vi "magnetic-actuator.vi"() -> ()   [LabVIEW 2021]
uses:
  mag-settings.ctl
panel:
  in  "On":bool
  in  "Off":bool
  out "Cycle Running":bool
  out "Last Command Sent":string
  out "Countdown Timer (mS)":u32
  out "last event":u32
  out "Coil Active":bool
  in  "Stop Cycle":bool
  in  "Start Cycle":bool
  in  "Eng Mode":bool
  out "LOW Cycle Time (Seconds)":dbl
  out "HIGH Cycle Time (Seconds)":dbl
  out "Duty %":dbl
  in  "Reflux Ratio":dbl
  in  "Period (Seconds)":dbl=5.0
  in  "Exit Program":bool
  # "TODO: CHANGE CYCLE TIME DISPLAY"
  # "TODO: MAKE THIS AESTHETIC"
  # "HIGH Cycle = period*(1/Duty Cycle)"
  # "Manual Controls"
  # "LOW Cycle = period - HIGH Cycle Time"
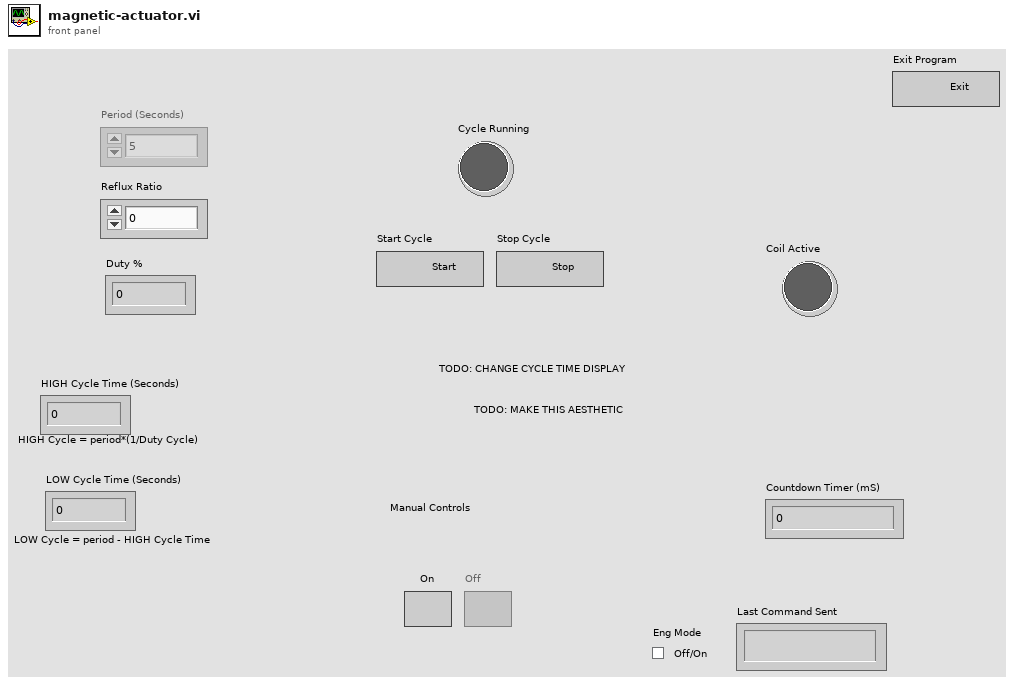
[diagram p1: front panel]
types:
  T1 = typedef "mag-settings.ctl" = cluster{"COM Port (COM10)":refnum<visa-resource-name>, "ADAM-ID":dbl, "ADAM-DO-channel":dbl, "Period (Seconds)":dbl, "Duty Cycle":dbl, "Eng Mode":bool}
  T2 = enum8{"Enabled", "Disabled", "Disabled and Grayed Out"}
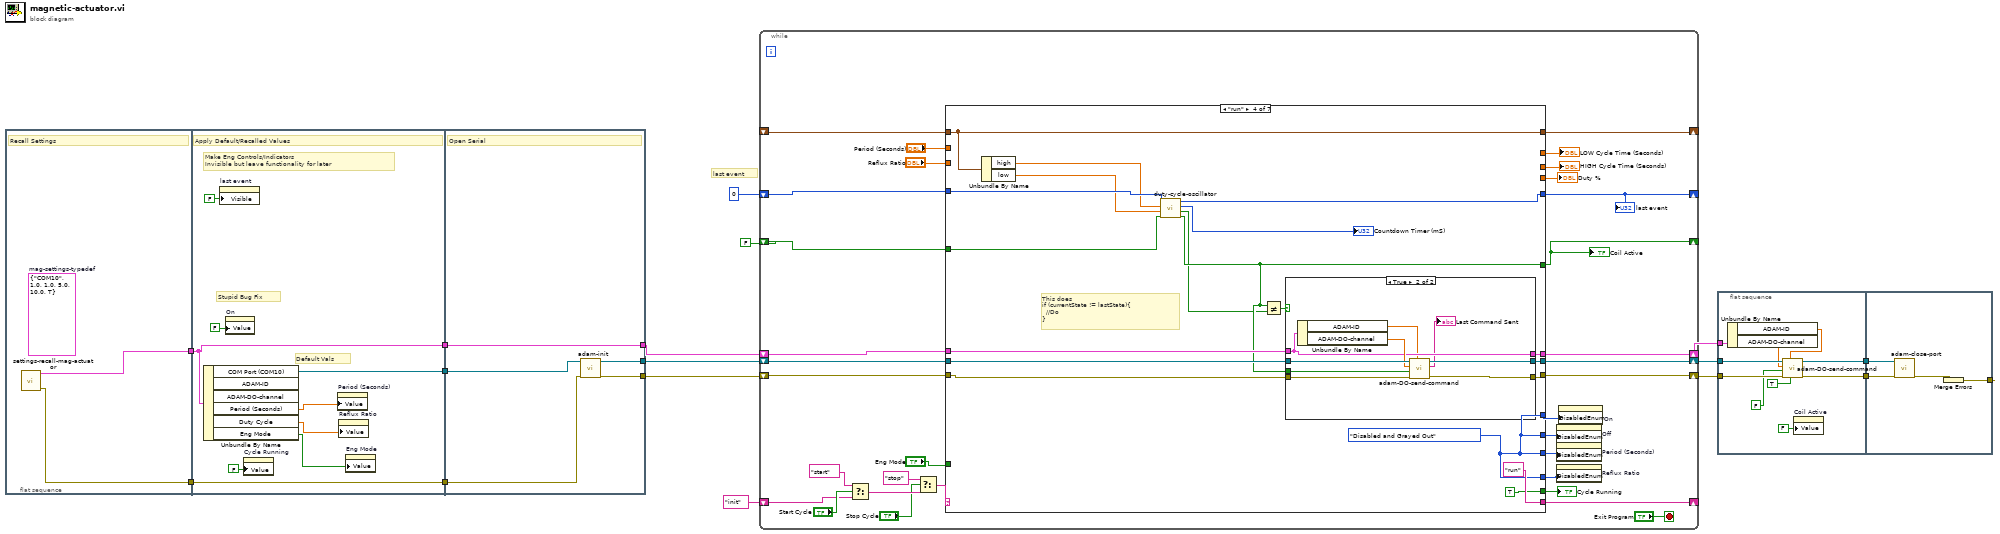
[diagram p0: block diagram]
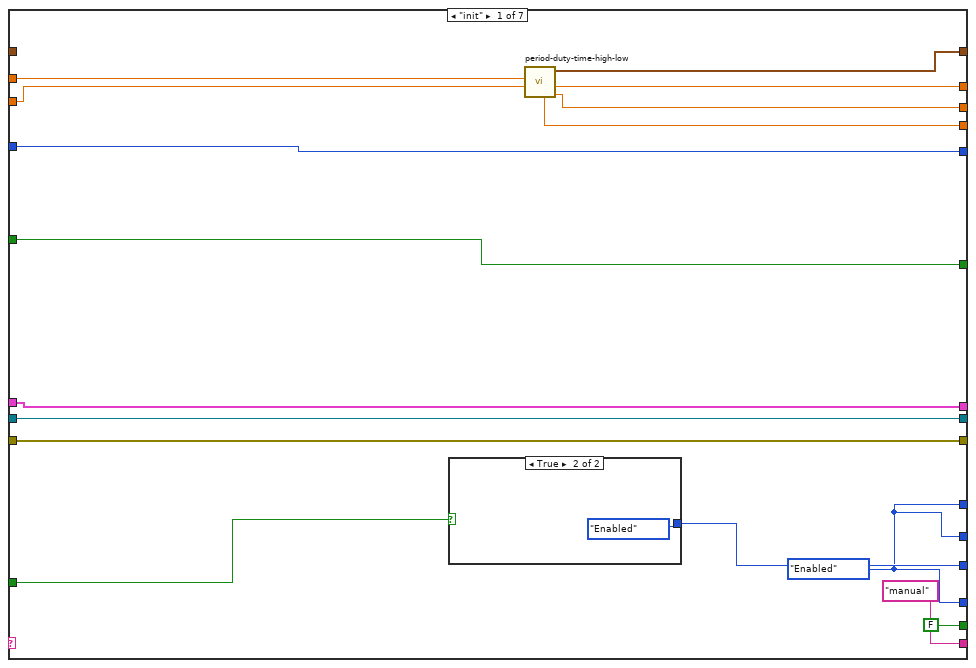
[diagram p2: hidden frame]
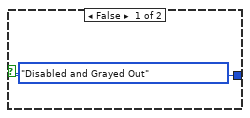
[diagram p3: hidden frame]
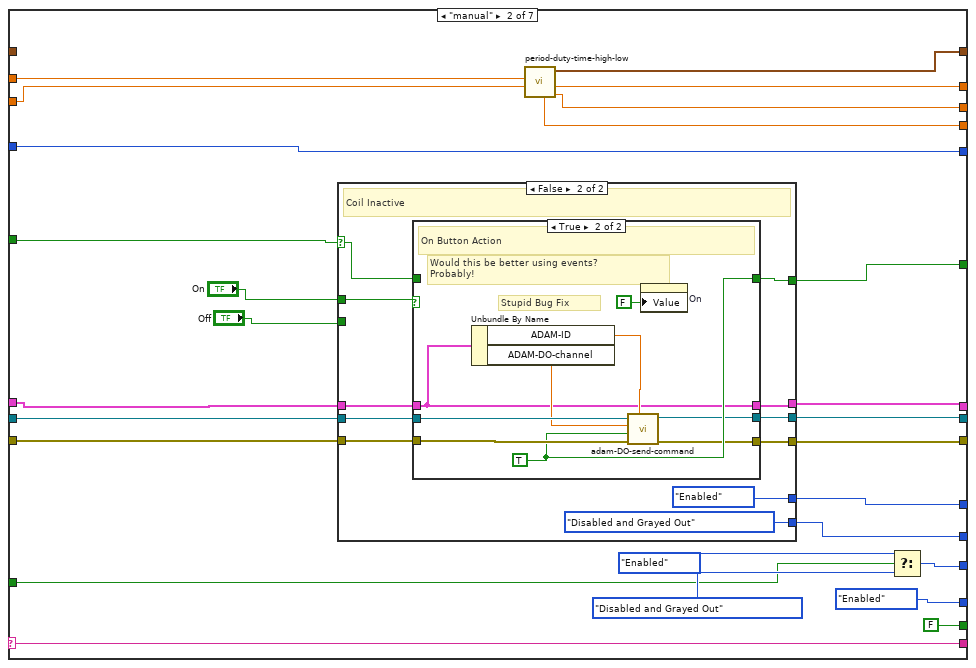
[diagram p4: hidden frame]
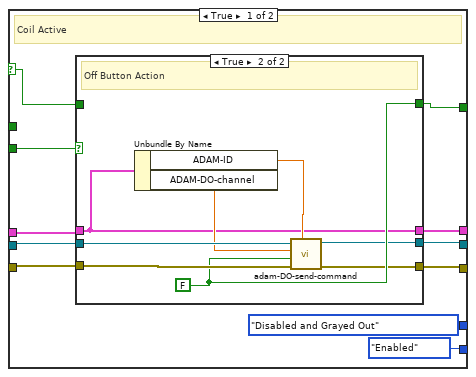
[diagram p5: hidden frame]
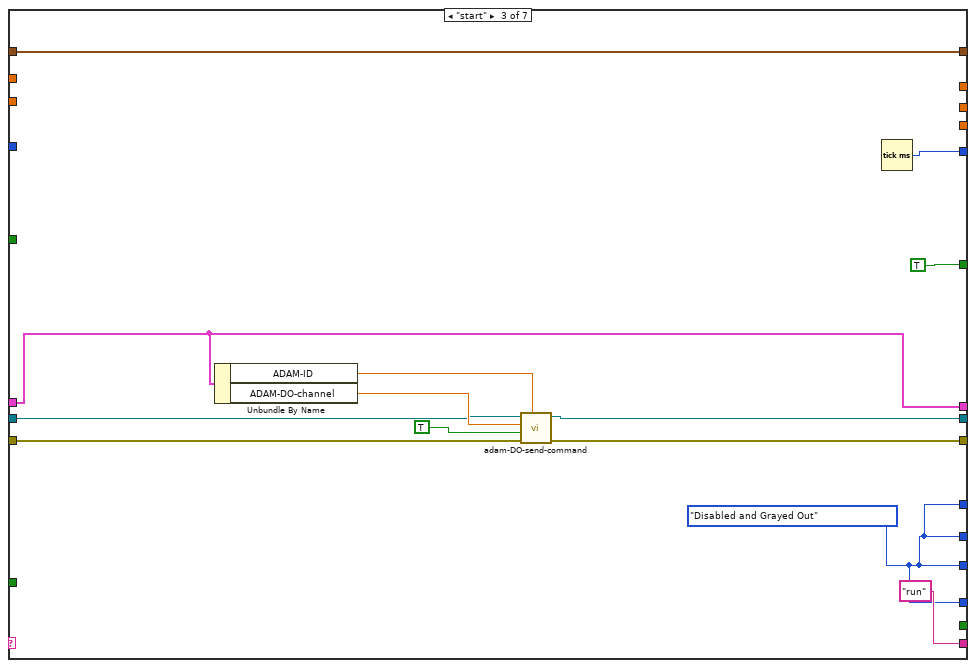
[diagram p8: hidden frame]
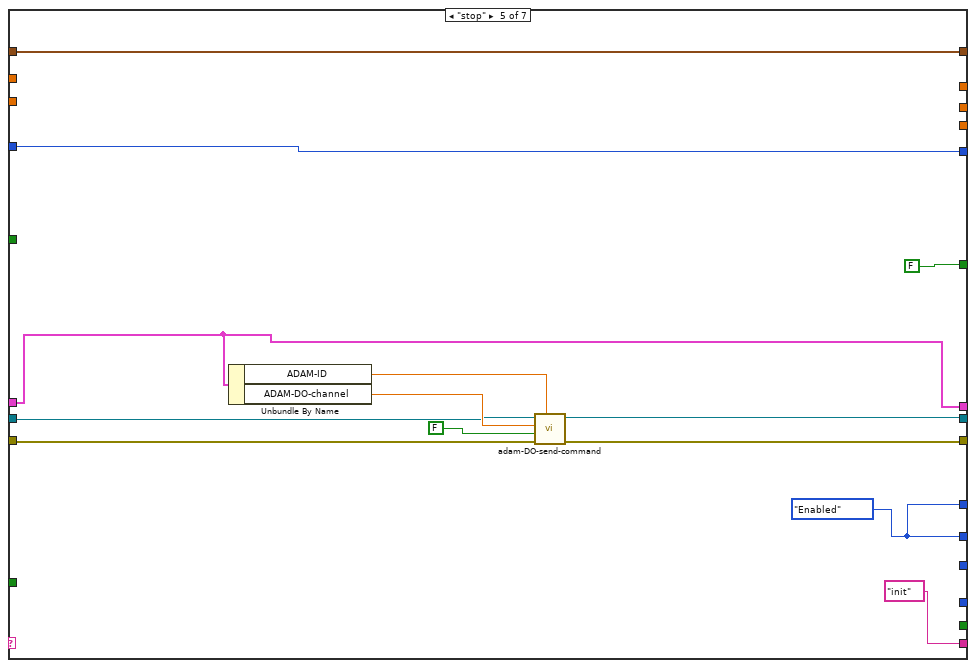
[diagram p10: hidden frame]
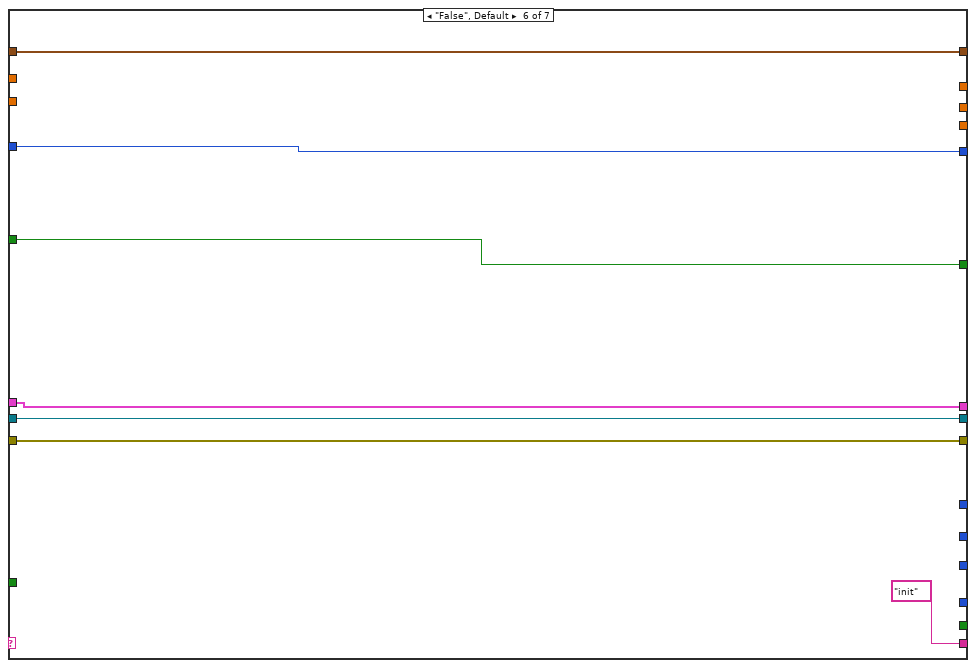
[diagram p11: hidden frame]
diagram:
  # "last event"
  n1 = flat-sequence {
    tunnel: [w18] -> w13
    tunnel: [w17] -> w5
    tunnel: [w27] -> w14
    tunnel: w13 -> [w26]
    tunnel: [w26] -> w12
    tunnel: w5 -> [w25]
    tunnel: [w25] -> w4
    tunnel: [w32] -> w11
    tunnel: [w31] -> w10
    tunnel: w14 -> [w29]
    tunnel: w12 -> [w30]
    tunnel: [w28] -> w3
    tunnel: w4 -> [w28]
    frame #0 {
      (unwired) T1 {"COM Port (COM10)"="COM10", "ADAM-ID"=1.0, "ADAM-DO-channel"=1.0, "Period (Seconds)"=5.0, "Duty Cycle"=10.0, "Eng Mode"=TRUE}  # mag-settings-typedef
      # "Recall Settings"
      n2 = call "settings-recall-mag-actuator.vi"() -> ("error out"=w18:errorcluster, "mag-settings"=w17:T1)  [unwired: 9 in, 1 out]
    }
    frame #1 {
      # "Default Vals"
      # "Make Eng Controls/Indicators\nInvisible but leave functionality for later"
      # "Stupid Bug Fix"
      # "Apply Default/Recalled Values"
      n3 = Unbundle By Name(w25) -> ("COM Port (COM10)"=w27:refnum<visa-resource-name>, "Period (Seconds)"=w24:dbl, "Duty Cycle"=w23:dbl, "Eng Mode"=w22:bool)  [unwired: 2 out]
      n4 = property on="last event" class="DigNum (strict)"("Visible"=FALSE) -> ()  [unwired: 2 in, 2 out]
      n5 = property on="On" class="Bool (strict)"("Value"=FALSE ("On")) -> ()  [unwired: 2 in, 2 out]
      n6 = property on="Cycle Running" class="Bool (strict)"("Value"=FALSE ("Running")) -> ()  [unwired: 2 in, 2 out]
      n7 = property on="Period (Seconds)" class="DigNum (strict)"("Value"=w24) -> ()  [unwired: 2 in, 2 out]
      n8 = property on="Reflux Ratio" class="DigNum (strict)"("Value"=w23) -> ()  [unwired: 2 in, 2 out]
      n9 = property on="Eng Mode" class="Bool (strict)"("Value"=w22) -> ()  [unwired: 2 in, 2 out]
    }
    frame #2 {
      # "Open Serial"
      n10 = call "adam-init.vi"("error in (no error)"=w30, "COM Port (COM10)"=w29) -> ("error out"=w31:errorcluster, "VISA resource name out"=w32:refnum<visa-resource-name>)  [unwired: 8 in]
    }
  }
  n11 = while {
    shift-right: [w58] -> _
    shift-left: "init" -> [w36]
    shift-right: [w57] -> _
    shift-left: u32 0 ("millisecond timer value") -> [w56]
    shift-right: [w55] -> _
    shift-left: _ -> [w54]
    shift-right: [w51] -> _
    shift-left: FALSE ("t") -> [w50]
    shift-right: [w47] -> w7
    shift-left: w11 -> [w46]
    shift-right: [w45] -> w6
    shift-left: w10 -> [w44]
    shift-right: [w41] -> w2
    shift-left: w3 -> [w42]
    stop <- "Exit Program" stop-if-true
    n12 = Select(t="start", s="Start Cycle", f=w36) -> (s? t:f=w49:string)
    n13 = Select(t="stop", s="Stop Cycle", f=w49) -> (s? t:f=w61:string)
    n14 = case shown="\"run\"" w61 {
      selector: w61 -> [_ w108 _ _ _ _ w223]
      tunnel: "Period (Seconds)" -> [w75 w106 _ _ _ _ _]
      tunnel: ["manual" w108 "run" "run" "init" "init" w223] -> w58
      tunnel: [w73 w104 w167 w186 w210 w219 w225] -> w57
      tunnel: w56 -> [w73 w104 _ w171 w210 w219 w225]
      tunnel: [w76 w107 w166 w180 w209 w218 w226] -> w55
      tunnel: w54 -> [_ _ w166 w180 w209 w218 w226]
      tunnel: [w79 w98 w156 w176 _ _ _] -> w53
      tunnel: "Eng Mode" -> [w80 w95 _ _ _ _ _]
      tunnel: [w68 T2."Enabled" ("Disabled") w156 w176 _ _ _] -> w52
      tunnel: [w70 w91 TRUE ("t") w173 FALSE ("t") w213 w224] -> w51
      tunnel: w50 -> [w70 w101 _ w174 _ w213 w224]
      tunnel: [w78 w90 w158 w184 w202 w216 w222] -> w47
      tunnel: w46 -> [w78 w92 w159 w183 w203 w216 w222]
      tunnel: [w77 w89 w157 w182 w201 w215 w221] -> w45
      tunnel: w44 -> [w77 w94 w163 w181 w204 w215 w221]
      tunnel: "Reflux Ratio" -> [w74 w105 _ _ _ _ _]
      tunnel: w42 -> [w72 w93 w164 w179 w205 w214 w220]
      tunnel: [w72 w88 w164 w178 w205 w214 w220] -> w41
      tunnel: [FALSE ("Running") FALSE ("Running") _ TRUE ("Running") _ _ _] -> w40
      tunnel: [w68 w100 w156 w176 w200 _ _] -> w39
      tunnel: [w68 w99 w156 w176 w200 _ _] -> w38
      tunnel: [w67 w87 _ _ _ _ _] -> w35
      tunnel: [w66 w86 _ _ _ _ _] -> w34
      tunnel: [w65 w85 _ _ _ _ _] -> w33
      frame "init" {
        w68 = T2."Enabled" ("Disabled")
        n15 = case shown="True" w80 {
          tunnel: [T2."Disabled and Grayed Out" ("Disabled") T2."Enabled" ("Disabled")] -> w79
          frame False {
          }
          frame True {
          }
        }
        n16 = call "period-duty-time-high-low.vi"("Duty Cycle"=w74, "Period (Seconds)"=w75) -> ("Time High (Seconds)"=w66:dbl, "Time Low (Seconds)"=w67:dbl, "delaytimes mS"=w76:cluster{"low":dbl, "high":dbl}, "Duty %"=w65:dbl)  [unwired: 6 in]
      }
      frame "manual" {
        n17 = case shown="False" w101 {
          selector: w101 -> [w116 w133]
          tunnel: [T2."Enabled" ("Disabled") T2."Disabled and Grayed Out" ("Disabled")] -> w100
          tunnel: [T2."Disabled and Grayed Out" ("Disabled") T2."Enabled" ("Disabled")] -> w99
          tunnel: "On" -> [_ w140]
          tunnel: w94 -> [w111 w139]
          tunnel: w93 -> [w110 w138]
          tunnel: w92 -> [w112 w137]
          tunnel: [w115 w136] -> w91
          tunnel: [w114 w135] -> w90
          tunnel: [w113 w134] -> w89
          tunnel: "Off" -> [w117 _]
          tunnel: [w109 w132] -> w88
          frame True {
            # "Coil Active"
            n18 = case shown="True" w117 {
              tunnel: w111 -> [w120 w131]
              tunnel: w110 -> [w122 w124]
              tunnel: w112 -> [w121 w130]
              tunnel: [w123 w129] -> w115
              tunnel: [w121 w128] -> w114
              tunnel: [w120 w127] -> w113
              tunnel: w116 -> [w123 _]
              tunnel: [w122 w124] -> w109
              frame False {
              }
              frame True {
                w129 = FALSE ("Channel Active")
                # "Off Button Action"
                n19 = Unbundle By Name(w124) -> ("ADAM-ID"=w126:dbl, "ADAM-DO-channel"=w125:dbl)
                n20 = call "adam-DO-send-command.vi"("Device Address"=w126, "error in (no error)"=w131, "Channel Active"=w129, "Channel Number"=w125, "VISA Refnum in"=w130) -> ("error out"=w127:errorcluster, "VISA Refnum out"=w128:refnum<visa-resource-name>)  [unwired: 1 in, 4 out]
              }
            }
          }
          frame False {
            # "Coil Inactive"
            n21 = case shown="True" w140 {
              tunnel: w139 -> [w143 w155]
              tunnel: w138 -> [w145 w148]
              tunnel: w137 -> [w144 w154]
              tunnel: [w146 w153] -> w136
              tunnel: [w144 w152] -> w135
              tunnel: [w143 w151] -> w134
              tunnel: w133 -> [w146 _]
              tunnel: [w145 w148] -> w132
              frame False {
              }
              frame True {
                w153 = TRUE ("Channel Active")
                # "Stupid Bug Fix"
                # "Would this be better using events?\nProbably!"
                # "On Button Action"
                n22 = Unbundle By Name(w148) -> ("ADAM-ID"=w150:dbl, "ADAM-DO-channel"=w149:dbl)
                n23 = call "adam-DO-send-command.vi"("Device Address"=w150, "error in (no error)"=w155, "Channel Active"=w153, "Channel Number"=w149, "VISA Refnum in"=w154) -> ("error out"=w151:errorcluster, "VISA Refnum out"=w152:refnum<visa-resource-name>)  [unwired: 1 in, 4 out]
                n24 = property on="On" class="Bool (strict)"("Value"=FALSE ("On")) -> ()  [unwired: 2 in, 2 out]
              }
            }
          }
        }
        n25 = call "period-duty-time-high-low.vi"("Duty Cycle"=w105, "Period (Seconds)"=w106) -> ("Time High (Seconds)"=w86:dbl, "Time Low (Seconds)"=w87:dbl, "delaytimes mS"=w107:cluster{"low":dbl, "high":dbl}, "Duty %"=w85:dbl)  [unwired: 6 in]
        n26 = Select(t=T2."Enabled" ("Disabled"), s=w95, f=T2."Disabled and Grayed Out" ("Disabled")) -> (s? t:f=w98:T2)
      }
      frame "start" {
        w156 = T2."Disabled and Grayed Out" ("Disabled")
        n27 = Unbundle By Name(w164) -> ("ADAM-ID"=w161:dbl, "ADAM-DO-channel"=w162:dbl)
        n28 = call "adam-DO-send-command.vi"("Device Address"=w161, "error in (no error)"=w163, "Channel Active"=TRUE, "Channel Number"=w162, "VISA Refnum in"=w159) -> ("error out"=w157:errorcluster, "VISA Refnum out"=w158:refnum<visa-resource-name>)  [unwired: 1 in, 4 out]
        n29 = Tick Count (ms)() -> (millisecond timer value=w167:u32)
      }
      frame "run" {
        w176 = T2."Disabled and Grayed Out" ("Disabled")
        # "This does\nif (currentState != lastState){\n  //Do\n}"
        n30 = Unbundle By Name(w180) -> ("high"=w170:dbl, "low"=w169:dbl)
        n31 = call "duty-cycle-oscillator.vi"("Input State"=w174, "time low mS"=w169, "time high mS"=w170, "lastEvent mS"=w171) -> ("output state"=w173:bool, "lastState"=w172:bool, "Countdown Timer (mS)"=→"Countdown Timer (mS)":u32, "lastEvent ms Out"=w186:u32)  [unwired: 4 in]
        n32 = Not Equal?(x=w173, y=w172) -> (x != y?=w185:bool)
        n33 = case shown="True" w185 {
          tunnel: [w190 w196] -> w184
          tunnel: w183 -> [w190 w198]
          tunnel: [w189 w195] -> w182
          tunnel: w181 -> [w189 w197]
          tunnel: w179 -> [w188 w193]
          tunnel: [w188 w193] -> w178
          tunnel: w173 -> [_ w199]
          frame False {
          }
          frame True {
            n34 = Unbundle By Name(w193) -> ("ADAM-ID"=w192:dbl, "ADAM-DO-channel"=w194:dbl)
            n35 = call "adam-DO-send-command.vi"("Device Address"=w192, "error in (no error)"=w197, "Channel Active"=w199, "Channel Number"=w194, "VISA Refnum in"=w198) -> ("error out"=w195:errorcluster, "command"=→"Last Command Sent":string, "VISA Refnum out"=w196:refnum<visa-resource-name>)  [unwired: 1 in, 3 out]
          }
        }
      }
      frame "stop" {
        w200 = T2."Enabled" ("Disabled")
        n36 = Unbundle By Name(w205) -> ("ADAM-ID"=w207:dbl, "ADAM-DO-channel"=w208:dbl)
        n37 = call "adam-DO-send-command.vi"("Device Address"=w207, "error in (no error)"=w204, "Channel Active"=FALSE, "Channel Number"=w208, "VISA Refnum in"=w203) -> ("error out"=w201:errorcluster, "VISA Refnum out"=w202:refnum<visa-resource-name>)  [unwired: 1 in, 4 out]
      }
      frame "False", Default {
      }
      frame "True" {
      }
    }
    "Coil Active" <- w51
    "last event" <- w57
    "Cycle Running" <- w40
    "Duty %" <- w33
    "HIGH Cycle Time (Seconds)" <- w34
    "LOW Cycle Time (Seconds)" <- w35
    n38 = property on="Off" class="Bool"("DisabledEnum"=w39) -> ()  [unwired: 2 in, 2 out]
    n39 = property on="Period (Seconds)" class="DigNum (strict)"("DisabledEnum"=w53) -> ()  [unwired: 2 in, 2 out]
    n40 = property on="Reflux Ratio" class="DigNum (strict)"("DisabledEnum"=w52) -> ()  [unwired: 2 in, 2 out]
    n41 = property on="On" class="Bool (strict)"("DisabledEnum"=w38) -> ()  [unwired: 2 in, 2 out]
  }
  n42 = flat-sequence {
    tunnel: w6 -> [w236]
    tunnel: w7 -> [w232]
    tunnel: [w235] -> w9
    tunnel: [w233] -> w8
    tunnel: w2 -> [w230]
    tunnel: w9 -> [w238]
    tunnel: w8 -> [w239]
    tunnel: [w237] -> _
    frame #0 {
      n43 = Unbundle By Name(w230) -> ("ADAM-ID"=w228:dbl, "ADAM-DO-channel"=w229:dbl)
      n44 = call "adam-DO-send-command.vi"("Stop All"=TRUE, "Device Address"=w228, "error in (no error)"=w236, "Channel Active"=FALSE, "Channel Number"=w229, "VISA Refnum in"=w232) -> ("error out"=w233:errorcluster, "VISA Refnum out"=w235:refnum<visa-resource-name>)  [unwired: 4 out]
      n45 = property on="Coil Active" class="Bool (strict)"("Value"=FALSE ("Coil Active")) -> ()  [unwired: 2 in, 2 out]
    }
    frame #1 {
      n46 = call "adam-close-port.vi"("error in (no error)"=w239, "VISA Refnum in"=w238) -> ("error out"=w240:errorcluster)  [unwired: 9 in]
      n47 = Merge Errors(w240) -> (w237:errorcluster)
    }
  }
